vi "Init Actor.vi"() -> (2 "Actor":refnum<class "Actor.lvclass">)   [LabVIEW 2025, in "_Template.lvlib" / "Templates.lvlib" / "TEMPLATE jettl Actor.lvlib"]
uses:
  TEMPLATE jettl Actor.lvlib
  jettl/jettl/Actor/Actor.lvclass
  TEMPLATE Actor/TEMPLATE Actor.lvlib
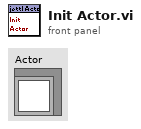
[diagram p1: front panel]
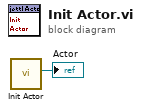
[diagram p0: block diagram]
diagram:
  n1 = call "Init Actor.vi"() -> ("Actor"=→"Actor":refnum<class "Actor.lvclass">)  [unwired: 11 in]
